vi "Name To Type.vi"(5 "Name":string) -> (2 "Type":string)   [LabVIEW 2019, in "Setting Database.lvclass"]
uses:
  Setting Database.lvclass
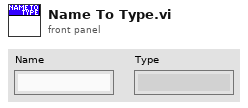
[diagram p1: front panel]
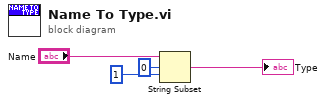
[diagram p0: block diagram]
diagram:
  n1 = String Subset(string="Name", offset (0)=0, length (rest)=1 ("length (rest)")) -> (substring=→"Type":string)
